vi "Parse Results From Answer.vi"(8 "error in (no error)":errorcluster, 11 "JSON":string) -> (0 "error out":errorcluster, 1 "data types of values":T1[](array[typedef]), 2 "JSON values":string[](array[string]), 3 "JSON keys":string[](array[string]), 5 "<JSON>":string caption="JSON.result")   [LabVIEW 2023, in "Communicator.lvclass"]
uses:
  Communicator.lvclass
  <vilib>/JDP Science/JSONtext/JSON Value Type.ctl
  <vilib>/JDP Science/JSONtext/Next JSON Value.vi
  <vilib>/JDP Science/JSONtext/String Subset.vi
  <vilib>/JDP Science/JSONtext/Parsing/Advance past next JSON Value (inlined COPY).vi
  <vilib>/JDP Science/JSONtext/Parsing/Advance past whitespace.vi
  <vilib>/JDP Science/JSONtext/Parsing/Advance past String.vi
  <vilib>/JDP Science/JSONtext/Parsing/Advance past Number.vi
  <vilib>/JDP Science/JSONtext/Parsing/Advance past Line Ending.vi
  <vilib>/JDP Science/JSONtext/Parsing/Parse Full Path or Item Name.vi
  <vilib>/JDP Science/JSONtext/Parsing/Advance past Array.vi
  <vilib>/JDP Science/JSONtext/Parsing/Advance past Object.vi
  <vilib>/JDP Science/JSONtext/support/Error Cluster From Code.vi
  <vilib>/JDP Science/JSONtext/Offset/Find Item Locations by Path.vi
  <vilib>/JDP Science/JSONtext/JSONtext.lvlib
panel:
  # "Connector Pane"
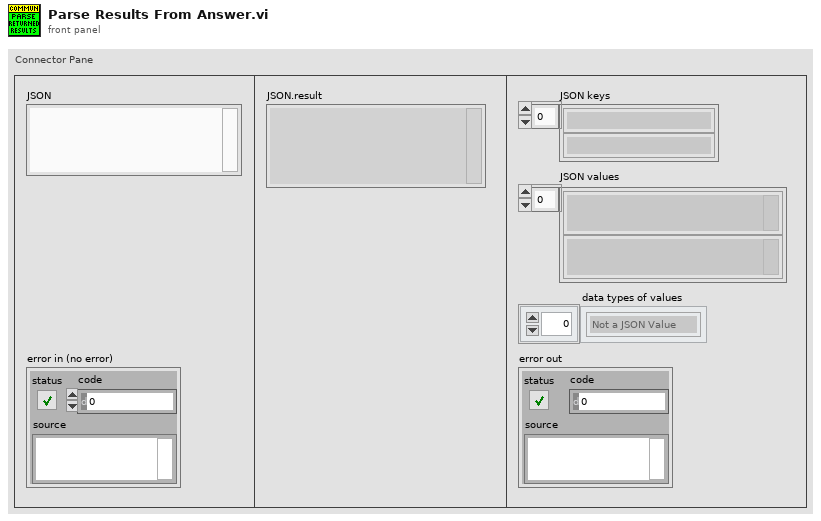
[diagram p1: front panel]
types:
  T1 = typedef "JSONtext.lvlib/JSON Value Type.ctl" = enum16{"Not a JSON Value", "JSON Object", "JSON Array", "String", "Number", "true", "false", "null"}
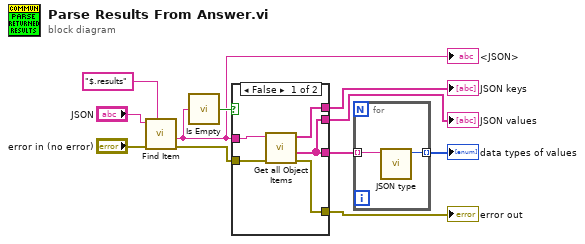
[diagram p0: block diagram]
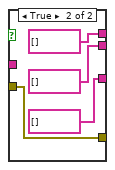
[diagram p2: hidden frame]
diagram:
  n1 = call <vilib>:"Find Item.vi"("$Path or Item Name"="$.results", "error in (no error)"="error in (no error)", "JSON"="JSON") -> ("error out"=w6:errorcluster, "<JSON>"=w4:string)  [unwired: 5 in, 2 out]
  "<JSON>" <- w4
  n2 = call <vilib>:"Is Empty.vi"("JSON"=w4) -> ("Empty"=w5:bool)  [unwired: 4 in]
  n3 = case shown="False" w5 {
    tunnel: [w13 string[] [] ("Item Names")] -> w11
    tunnel: [w12 string[] [] ("<JSON>")] -> w3
    tunnel: w4 -> [w16 _]
    tunnel: w6 -> [w15 w17]
    tunnel: [w14 w17] -> w1
    tunnel: [w12 string[] [] ("<JSON>")] -> w2
    frame False {
      n4 = call <vilib>:"Get all Object Items.vi"("error in (no error)"=w15, "JSON"=w16) -> ("error out"=w14:errorcluster, "<JSON>"=w12:string[], "Item Names"=w13:string[])  [unwired: 6 in, 1 out]
    }
    frame True {
    }
  }
  "JSON keys" <- w11
  "JSON values" <- w3
  "error out" <- w1
  n5 = for {
    tunnel: w2 -> [w22] mode=indexing
    tunnel: [w21] -> w10 mode=indexing
    n6 = call <vilib>:"JSON type.vi"("JSON"=w22) -> ("JSON Value Type"=w21:T1)  [unwired: 9 in, 1 out]
  }
  "data types of values" <- w10
